vi "Get System Name.vi"(8 "error in (no error)":errorcluster, 11 "XBox One Controller in":refnum<class "XBox One Controller.lvclass">) -> (0 "error out":errorcluster, 2 "System Name":string, 3 "XBox One Controller out":refnum<class "XBox One Controller.lvclass">)   [LabVIEW 2014, in "Xbox One Controller.lvlib" / "XBox One Controller.lvclass"]
uses:
  XBox One Controller.lvclass
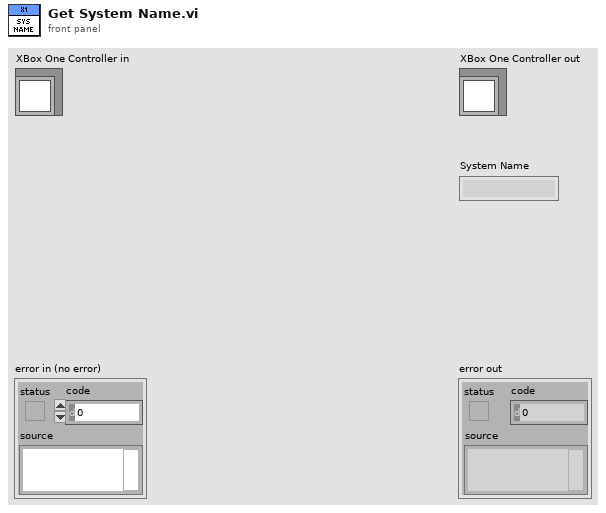
[diagram p1: front panel]
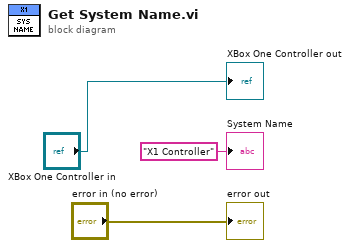
[diagram p0: block diagram]
diagram:
  "error out" <- "error in (no error)"
  "XBox One Controller out" <- "XBox One Controller in"
  "System Name" <- "X1 Controller" ("System Name")
